vi "Write Data Msg.vi"(10 "Data Msg":refnum<class "Data Msg.lvclass">, 11 "Registration Msg In":refnum<class "Registration Msg.lvclass">) -> (3 "Registration Msg Out":refnum<class "Registration Msg.lvclass">)   [LabVIEW 2016, in "Data Broadcasting.lvlib" / "Registration Msg.lvclass"]
doc: "-------------\nCopyright (c) 2013, Staab Engineering, a Texas Limited Liability Company\nAll rights reserved.\n\nRedistribution and use in source and binary forms, with or without modification, are permitted provided that the following conditions are met:\n\n1. Redistributions of source code must retain the above copyright notice, this list of conditions and the following disclaimer.\n2. Redistributions in binary form must reproduce the above copyright notice, this list of conditions and the following disclaimer in the documentation and/or other materials provided with the distribution.\n\nTHIS SOFTWARE IS PROVIDED BY THE COPYRIGHT HOLDERS AND CONTRIBUTORS \"AS IS\" AND ANY EXPRESS OR IMPLIED WARRANTIES, INCLUDING, BUT NOT LIMITED TO, THE IMPLIED WARRANTIES OF MERCHANTABILITY AND FITNESS FOR A PARTICULAR PURPOSE ARE DISCLAIMED. IN NO EVENT SHALL THE COPYRIGHT HOLDER OR CONTRIBUTORS BE LIABLE FOR ANY DIRECT, INDIRECT, INCIDENTAL, SPECIAL, EXEMPLARY, OR CONSEQUENTIAL DAMAGES (INCLUDING, BUT NOT LIMITED TO, PROCUREMENT OF SUBSTITUTE GOODS OR SERVICES; LOSS OF USE, DATA, OR PROFITS; OR BUSINESS INTERRUPTION) HOWEVER CAUSED AND ON ANY THEORY OF LIABILITY, WHETHER IN CONTRACT, STRICT LIABILITY, OR TORT (INCLUDING NEGLIGENCE OR OTHERWISE) ARISING IN ANY WAY OUT OF THE USE OF THIS SOFTWARE, EVEN IF ADVISED OF THE POSSIBILITY OF SUCH DAMAGE."
uses:
  <userlib>/_Frameworks/Staab/AF Data Broadcasting/Data Broadcasting/Registration Msg/Registration Msg.lvclass
  <userlib>/_Frameworks/Staab/AF Data Broadcasting/Data Broadcasting/Data Msg/Data Msg.lvclass
  <userlib>/_Frameworks/Staab/AF Data Broadcasting/Data Broadcasting/Registration Msg/Registration Msg.lvclass/Registration Msg.ctl
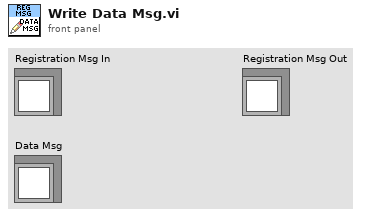
[diagram p1: front panel]
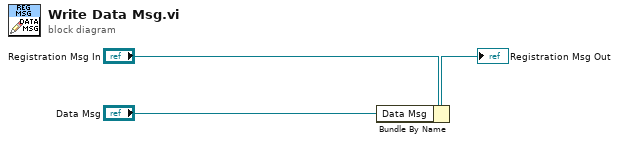
[diagram p0: block diagram]
diagram:
  n1 = Bundle By Name(cluster="Registration Msg In", "Data Msg"="Data Msg") -> (→"Registration Msg Out":refnum<class "Registration Msg.lvclass">)
